vi "运维调试_CODCr.vi"() -> ()   [LabVIEW 2016, in "CODCr库.lvlib"]
uses:
  <vilib>/Utility/miscctls.llb/LVPointTypeDef.ctl
  <vilib>/ptbypt/NI_PtbyPt.lvlib
  <vilib>/Utility/config.llb/NI_LVConfig.lvlib
panel:
  in  "仪器参数":bool
  in  "MB通信方式选择":enum16{"串口", "TCP"}(ring)
  in  "释放串口":bool
  in  "打开串口":bool
  in  "加标回收测试":bool
  in  "平行样测试":bool
  in  "定时启动":bool
  out "COM口":string
  in  "空白测试":bool
  in  "隐藏按钮":bool
  in  "写入消解温度时长":bool
  in  "保存KB值":bool
  in  "标样核查":bool
  out "启动时间":timestamp format="%<%Y/%m/%d %H:%M:%S>T"
  out "主循环次数":i32
  out "status":bool
  out "启动测量模式":T1(ring)
  out "曲线截距B":sgl format="%#_10g"
  out "曲线斜率K":sgl format="%#_10g"
  out "量程上限":sgl
  out "量程下限":sgl
  out "消解时长":u16
  out "消解温度":u16
  out "测量精度":u16
  out "测量结果":sgl
  out "标样参考值":sgl
  out "量程":u16
  out "工作状态":T1(ring)
  out "仪器时间":timestamp format="%<%X\n%x>T"
  out "关键参数区":T2
  out "状态告警区":T3
  out "测量数据区":T4 {"单位" items=["ug/L", "mg/L", "ppm", "mg/m3", "cm", "ppb", "ug/m3", "%", "nmol/mol", "umol/mol", "MPN/L", "MPN/100ml", "ng/m3", "NTU", "无量纲", "ms/cm", "us/cm", "℃", "mV", "万个/L"]}
  out "系统时间":timestamp format="%<%Y/%m/%d %H:%M:%S>T"
  in  "停止":bool
  in  "校时":bool
  in  "标样校准":bool
  in  "空白校准":bool
  in  "零点核查":bool
  in  "跨度核查":bool
  in  "水样测试":bool
  in  "返回":bool
  in  "设置":bool
  # "mg/L"
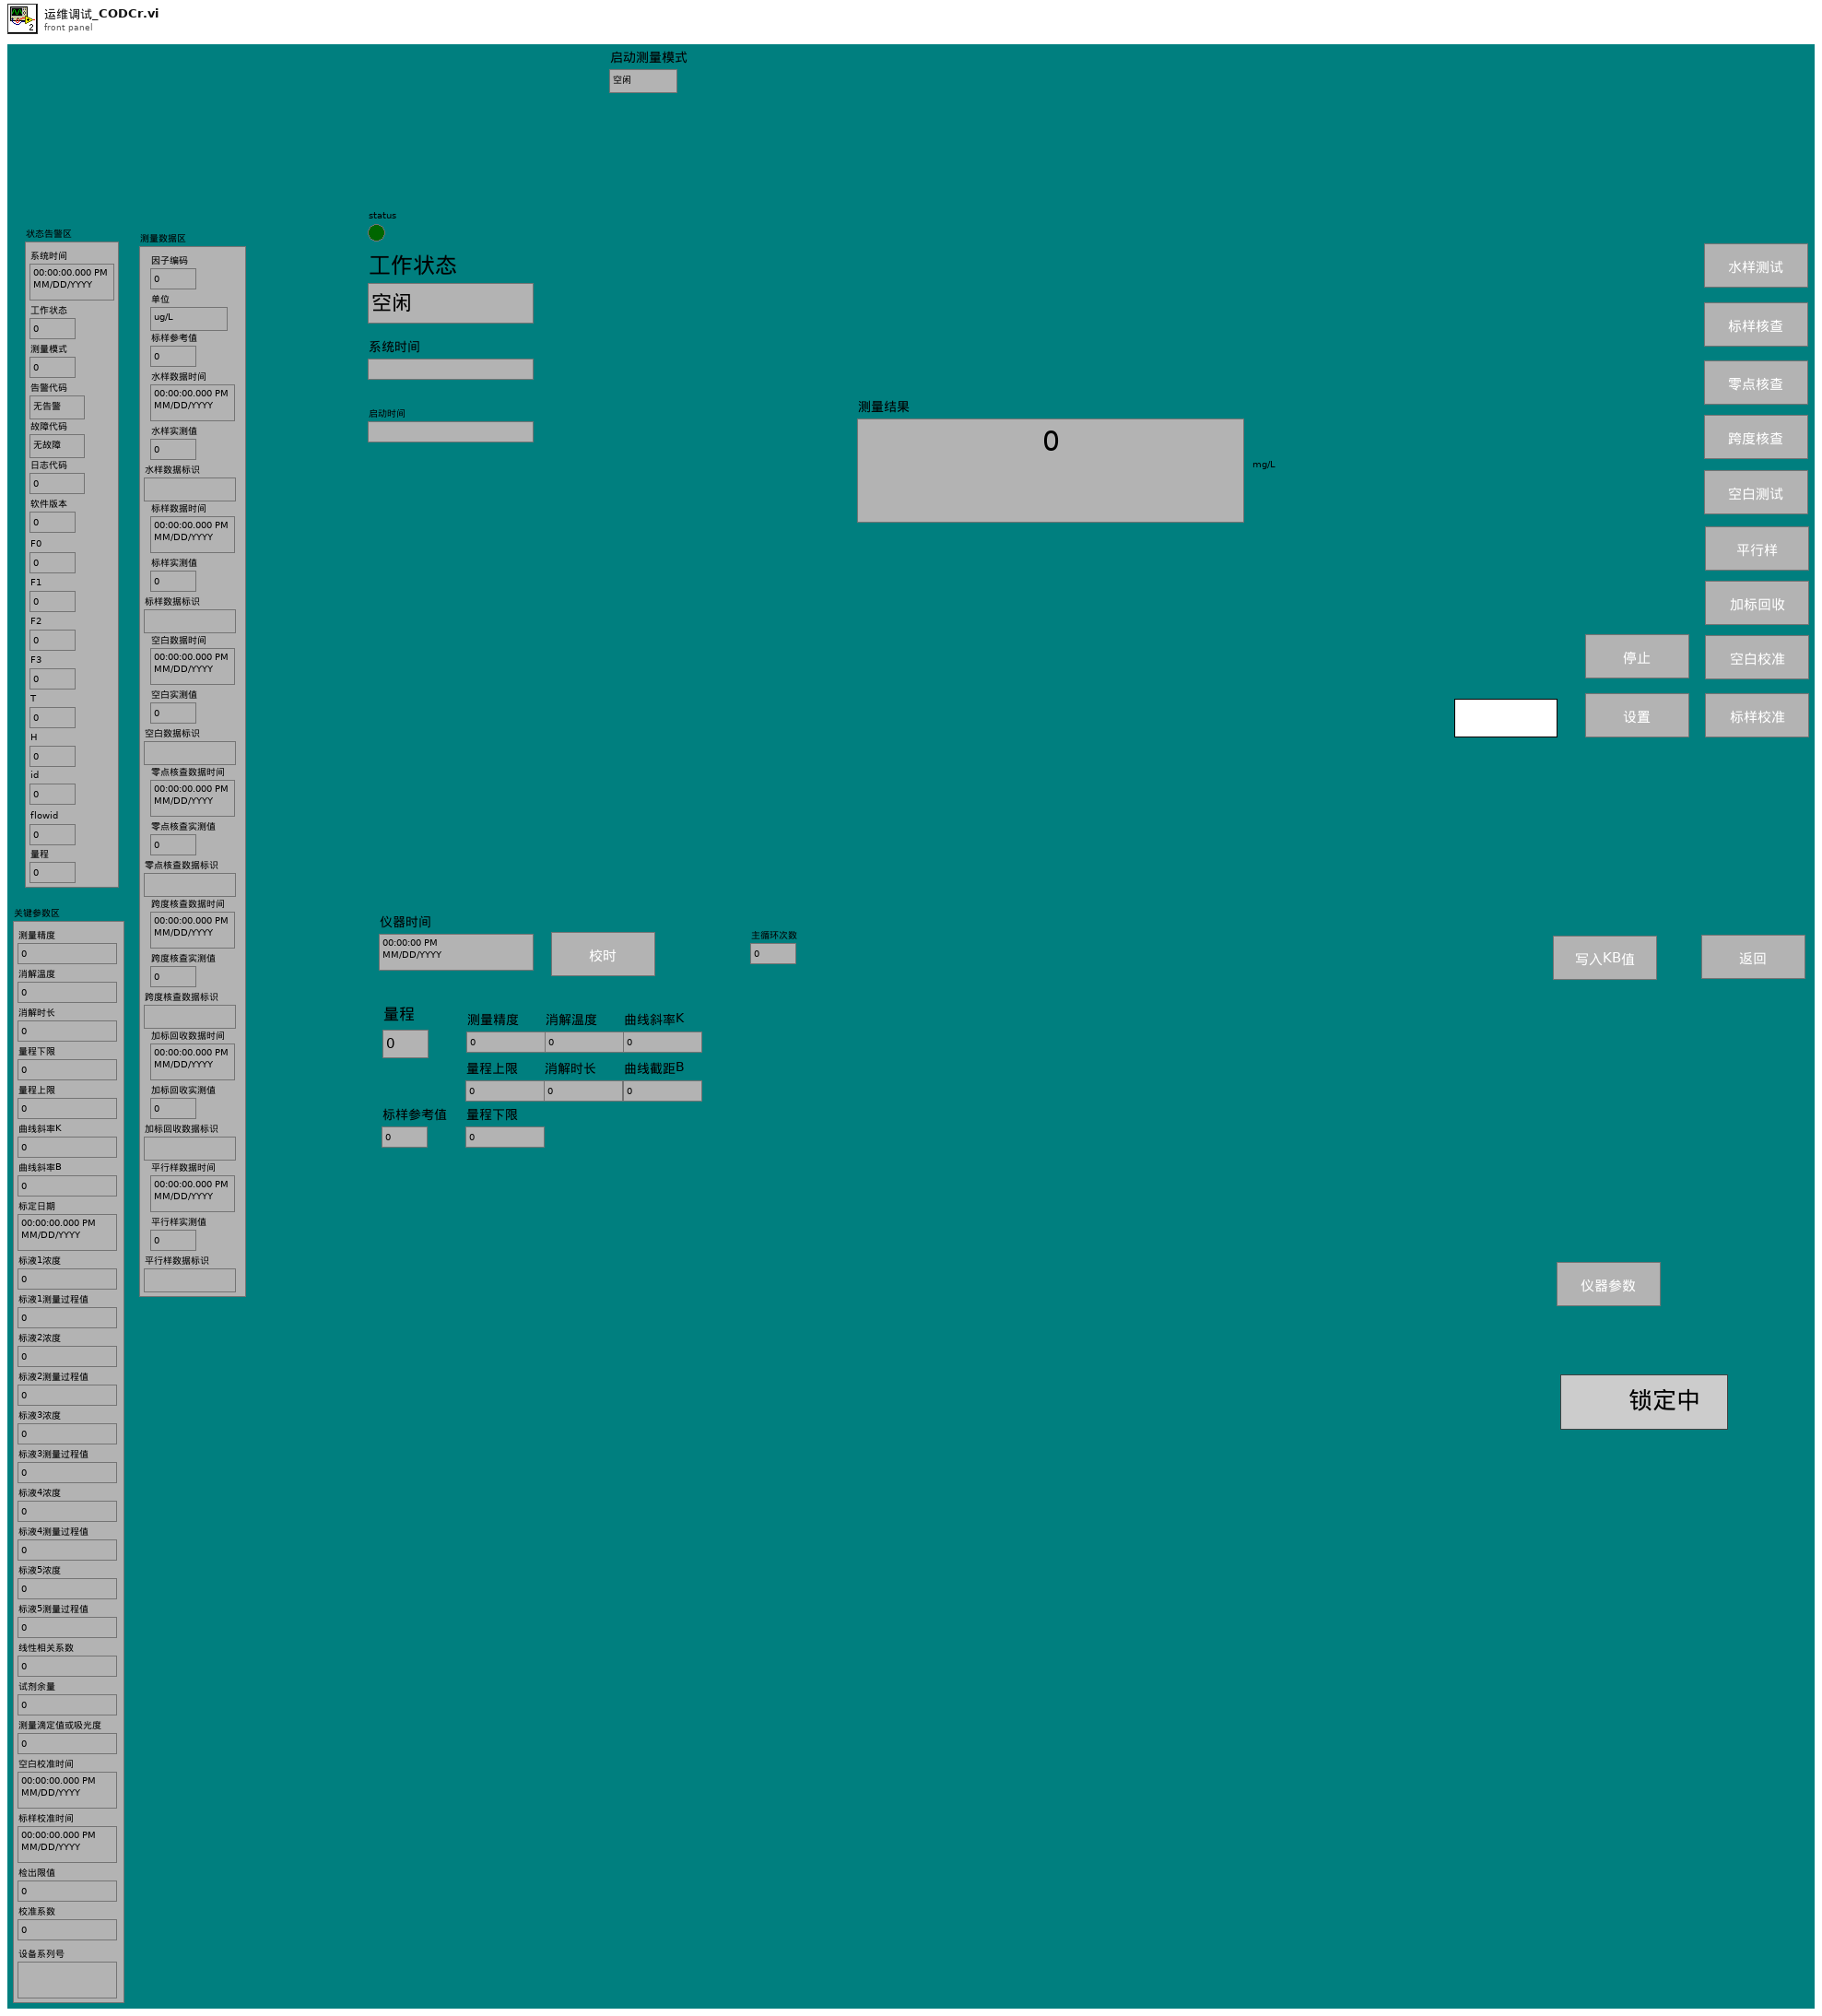
[diagram p1: front panel]
types:
  T1 = enum16{"空闲", "水样测试", "标样核查", "零点核查", "跨度核查", "空白测试", "平行样测试", "加标回收", "空白校准", "标样校准", "初始化（清洗）"}
  T2 = cluster{"测量精度":u16, "消解温度":u16, "消解时长":u16, "量程下限":sgl, "量程上限":sgl, "曲线斜率K":sgl, "曲线斜率B":sgl, "标定日期":timestamp, "标液1浓度":sgl, "标液1测量过程值":sgl, "标液2浓度":sgl, "标液2测量过程值":sgl, "标液3浓度":sgl, "标液3测量过程值":sgl, "标液4浓度":sgl, "标液4测量过程值":sgl, "标液5浓度":sgl, "标液5测量过程值":sgl, "线性相关系数":sgl, "试剂余量":u32, "测量滴定值或吸光度":sgl, "空白校准时间":timestamp, "标样校准时间":timestamp, "检出限值":sgl, "校准系数":sgl, "设备系列号":string}
  T3 = cluster{"系统时间":timestamp, "工作状态":u16, "测量模式":u16, "告警代码":enum16{"无告警", "缺试剂告警", "缺水样告警", "缺蒸馏水告警", "缺标液告警", "仪表漏液告警", "标定异常告警", "超量程告警", "加热异常", "低试剂预警", "超上限告警", "超下限告警", "仪表内部其他异常", "滴定异常告警", "电极异常告警", "量程切换告警", "参数设置告警", "PH电极电位异常", "电导率电极异常", "浊度光度异常", "溶解氧电极异常", "溶解氧光强异常", "温度异常告警", "PH异常告警", "溶解氧异常告警", "电导率异常告警", "浊度异常告警", "叶绿素异常告警", "藻密度异常告警", "蓝绿藻异常告警", "ORP异常告警", "氨氮异常告警", "清洁刷异常告警", "SD卡异常告警", "蓝牙异常告警", "Wifi异常告警", "流程异常告警"}, "故障代码":enum16{"无故障", "电机故障", "温度故障", "通讯故障", "滴定故障"}, "日志代码":u16, "软件版本":u16, "F0":sgl, "F1":sgl, "F2":sgl, "F3":sgl, "T":sgl, "H":sgl, "id":u16, "flowid":u16, "量程":u16}
  T4 = cluster{"因子编码":u32, "单位":u16, "标样参考值":sgl, "水样数据时间":timestamp, "水样实测值":sgl, "水样数据标识":string, "标样数据时间":timestamp, "标样实测值":sgl, "标样数据标识":string, "空白数据时间":timestamp, "空白实测值":sgl, "空白数据标识":string, "零点核查数据时间":timestamp, "零点核查实测值":sgl, "零点核查数据标识":string, "跨度核查数据时间":timestamp, "跨度核查实测值":sgl, "跨度核查数据标识":string, "加标回收数据时间":timestamp, "加标回收实测值":sgl, "加标回收数据标识":string, "平行样数据时间":timestamp, "平行样实测值":sgl, "平行样数据标识":string}
  T5 = cluster{"命令":string, "测量模式":enum16{"水样测量", "标样核查", "零点核查", "跨度核查", "空白测试", "加标回收", "平行样", "校零", "校标"}, "CODCr量程切换":enum32{"H", "L", "AUTO"}}
  T6 = typedef "LVPointTypeDef.ctl" = cluster{"Horizontal":i16, "Vertical":i16}
  T7 = typedef "NI_LVConfig.lvlib/Config Data RefNum.ctl" = refnum<k1>
  T8 = cluster{"运行模式":enum16{"维护模式", "常规模式", "应急模式", "质控模式"}}
  T9 = cluster{"时间标识":timestamp, "监测值":sgl, "单位":u16, "数据标识":string, "因子编码":u32, "标样参考值":sgl, "F0":sgl, "F1":sgl, "F2":sgl, "F3":sgl, "温度":sgl, "湿度":sgl, "量程标识":string, "LastTime":timestamp}
  T10 = cluster{"时间标识":timestamp, "设备":string, "日志信息":string}
  T11 = cluster{"时间标识":timestamp, "参数":string, "日志信息":string, "流程参数":string}
  T12 = enum16{"无告警", "缺试剂告警", "缺水样告警", "缺蒸馏水告警", "缺标液告警", "仪表漏液告警", "标定异常告警", "超量程告警", "加热异常", "低试剂预警", "超上限告警", "超下限告警", "仪表内部其他异常", "滴定异常告警", "电极异常告警", "量程切换告警", "参数设置告警", "PH电极电位异常", "电导率电极异常", "浊度光度异常", "溶解氧电极异常", "溶解氧光强异常", "温度异常告警", "PH异常告警", "溶解氧异常告警", "电导率异常告警", "浊度异常告警", "叶绿素异常告警", "藻密度异常告警", "蓝绿藻异常告警", "ORP异常告警", "氨氮异常告警", "清洁刷异常告警", "SD卡异常告警", "蓝牙异常告警", "Wifi异常告警", "流程异常告警"}
  T13 = cluster{"时间标识":timestamp, "设备":string, "日志信息":string, "流程参数":string}
  T14 = enum16{"水样测量", "标样核查", "零点核查", "跨度核查", "空白测试", "加标回收", "平行样", "校零", "校标"}
  T15 = cluster{"控制命令":enum16{"启动测量", "标样核查", "零点核查", "跨度核查", "空白测试", "平行样测试", "加标回收", "空白校准", "标样校准", "初始化（清洗）", "停止测试", "仪器重启", "校时", "模式设置", "测量间隔设置"}, "周期设置类型":enum16{"定点启动", "间隔启动"}, "定时功能启用":bool, "定时间隔":dbl, "24H周期设置":bool[], "零点核查时间":u16, "跨度核查时间":u16, "质控频次":enum16{"关闭", "每天", "星期一", "星期二", "星期三", "星期四", "星期五", "星期六", "星期日"}}
  T16 = cluster{"测量量程":dbl, "测量精度":dbl, "测量间隔":dbl, "消解温度":dbl, "消解时长":dbl, "空白校准时间":timestamp, "曲线截距":dbl, "曲线斜率":dbl, "测量检出限":dbl, "测量信号值":dbl, "线性相关系数":dbl, "二次多项式系数":dbl, "标样校准时间":timestamp, "稀释倍数":dbl, "三项式系数":dbl, "空白标定系数":dbl, "量程系数":dbl, "F0/ORPA":dbl, "F1/ORPB":dbl, "F2/ORPK":dbl, "F3":dbl, "F4":dbl, "F5":dbl, "F6":dbl, "F7":dbl, "X0/滴定数":dbl, "量程":dbl}
  T17 = cluster{"控制命令":enum16{"启动测量", "标样核查", "零点核查", "跨度核查", "空白测试", "平行样测试", "加标回收", "空白校准", "标样校准", "初始化（清洗）", "停止测试", "仪器重启", "校时", "模式设置", "测量间隔设置"}, "周期设置类型":enum16{"定点启动", "间隔启动"}, "定时功能启用":bool, "定时间隔":dbl, "24H周期设置":bool[], "空白核查时间":u16, "跨度核查时间":u16, "质控频次":enum16{"关闭", "每天", "星期一", "星期二", "星期三", "星期四", "星期五", "星期六", "星期日"}}
  T18 = cluster{"确定":bool, "测量量程":dbl, "测量精度":dbl, "测量间隔":dbl, "消解温度":dbl, "消解时长":dbl, "空白校准时间":timestamp, "曲线截距":dbl, "曲线斜率":dbl, "测量检出限":dbl, "测量信号值":dbl, "线性相关系数":dbl, "二次多项式系数":dbl, "标样校准时间":timestamp, "稀释倍数":dbl, "三项式系数":dbl, "空白标定系数":dbl, "量程系数":dbl, "F0/ORPA":dbl, "F1/ORPB":dbl, "F2/ORPK":dbl, "F3":dbl, "F4":dbl, "F5":dbl, "F6":dbl, "F7":dbl, "X0/滴定数":dbl, "量程":dbl}
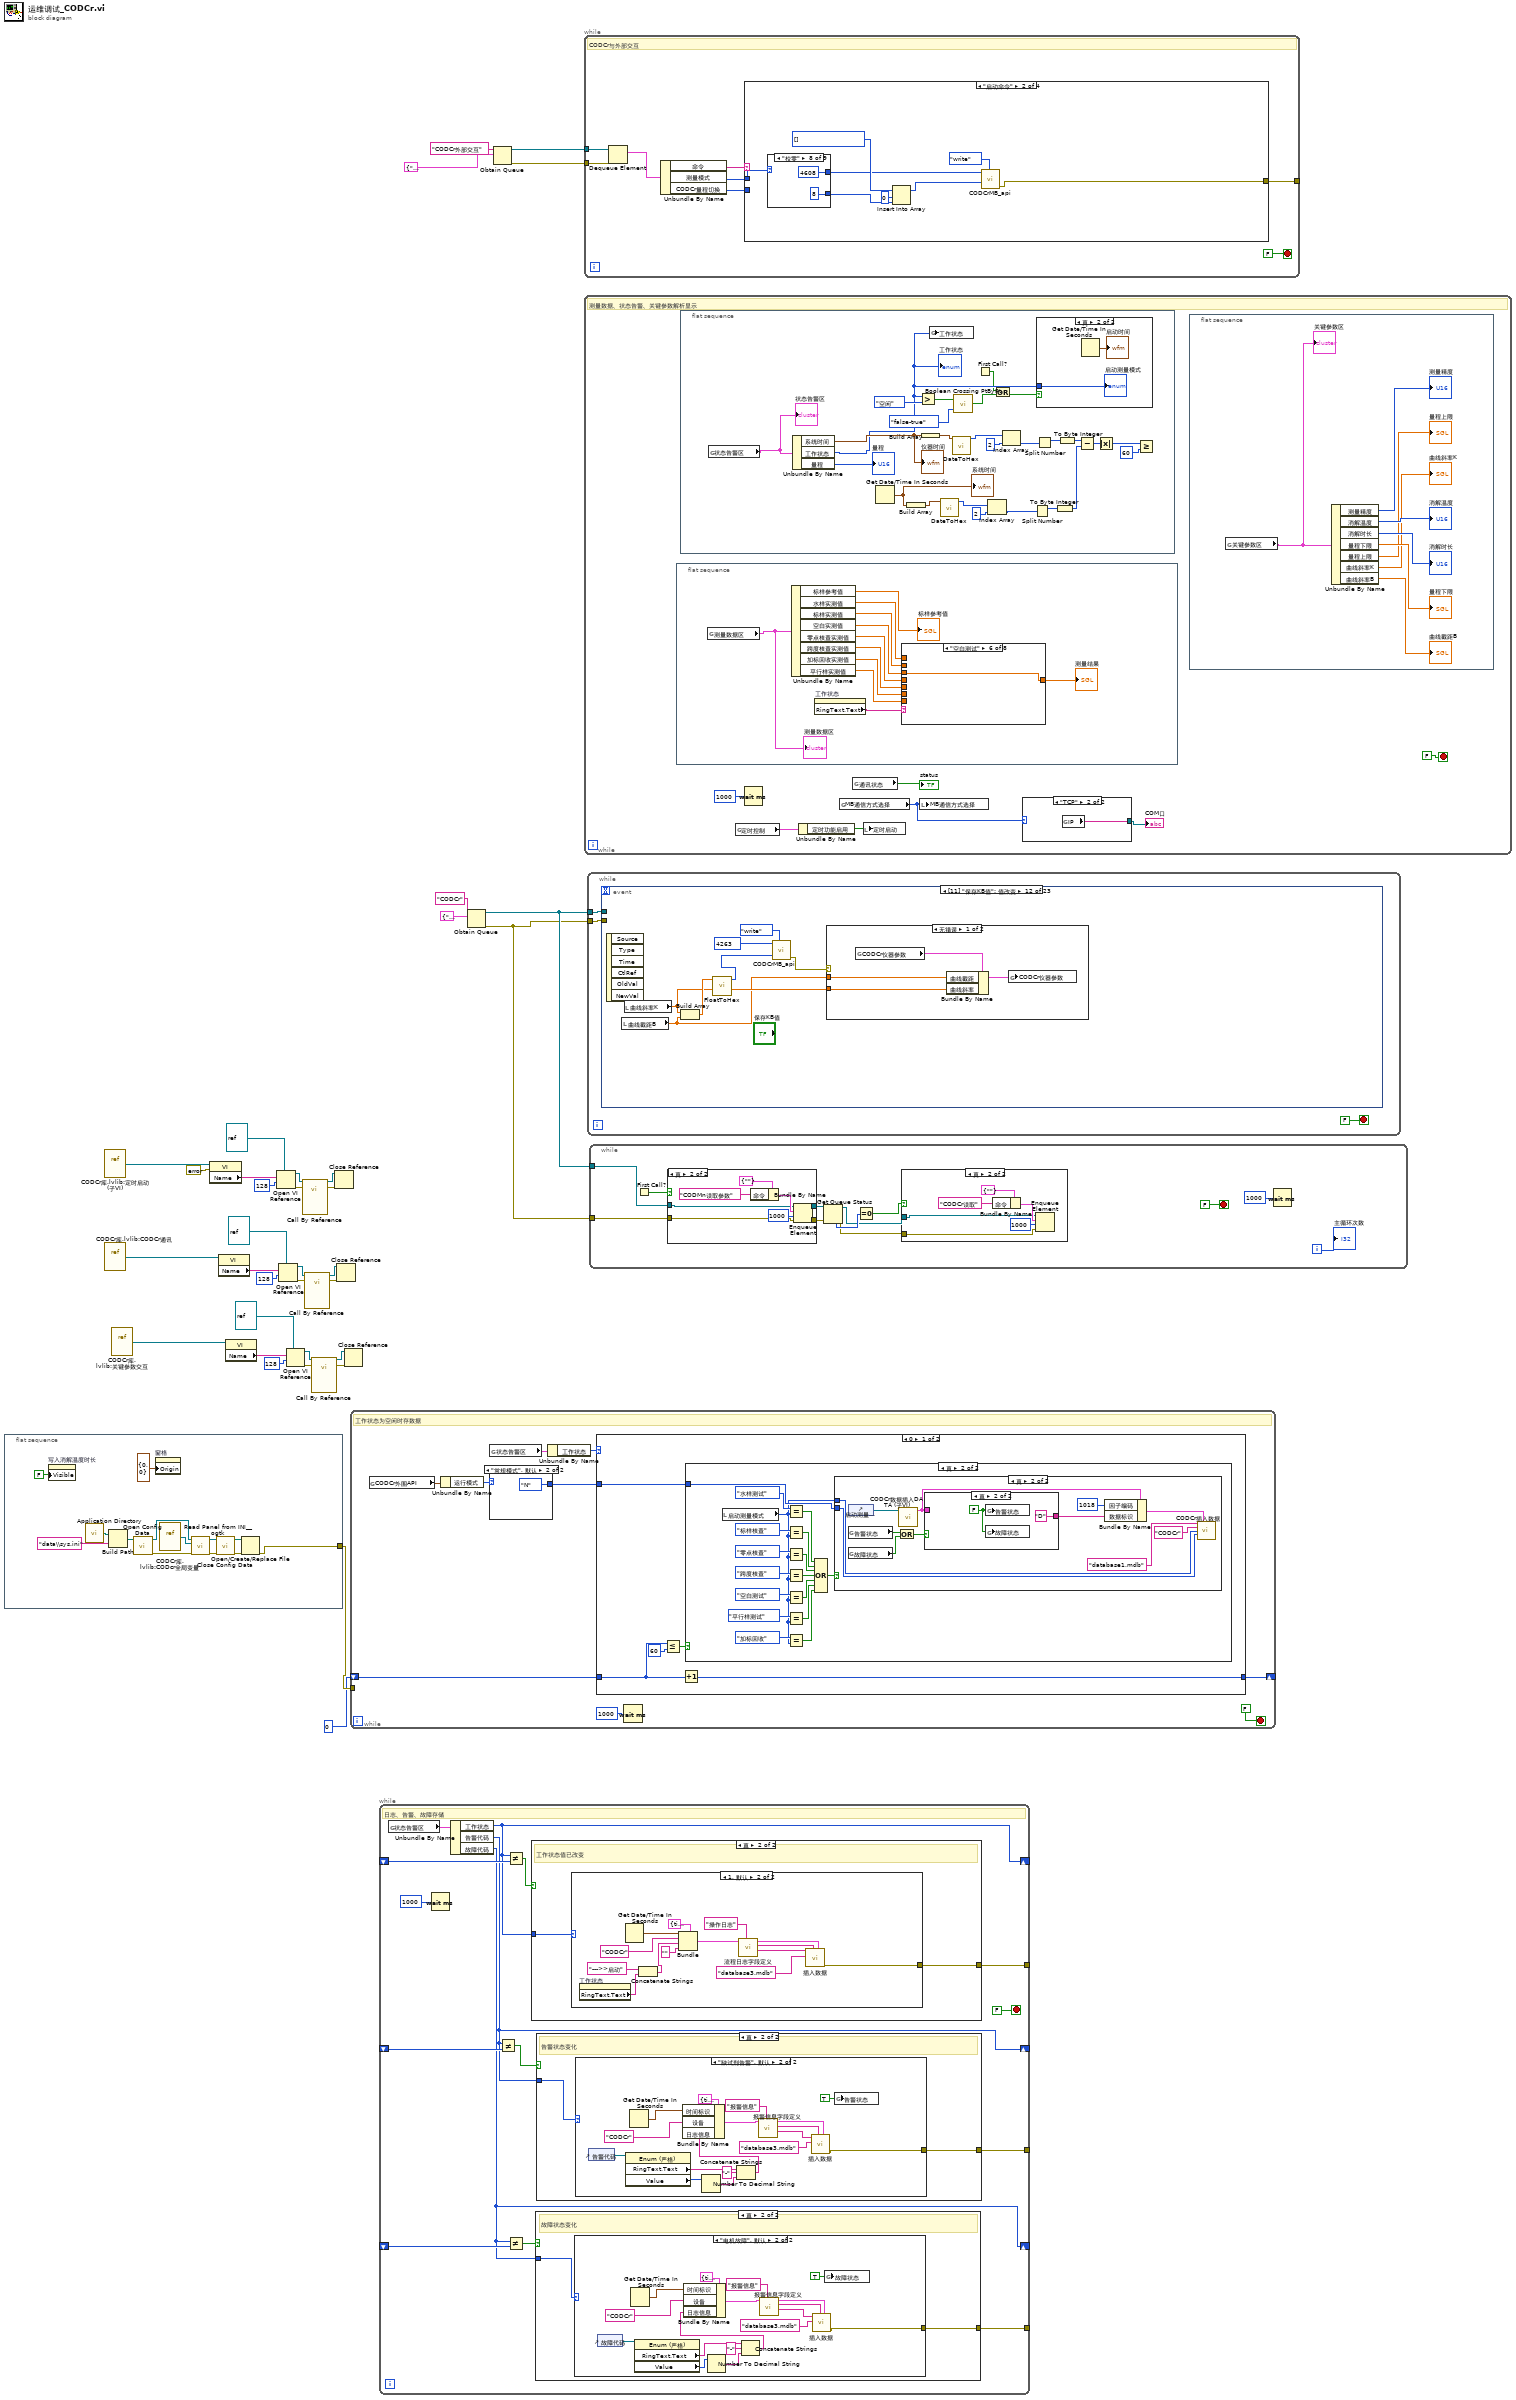
[diagram p0: block diagram]
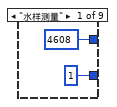
[diagram p5: hidden frame]
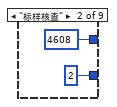
[diagram p6: hidden frame]
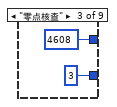
[diagram p7: hidden frame]
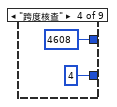
[diagram p8: hidden frame]
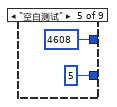
[diagram p9: hidden frame]
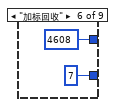
[diagram p10: hidden frame]
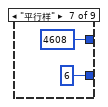
[diagram p11: hidden frame]
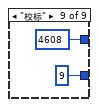
[diagram p12: hidden frame]
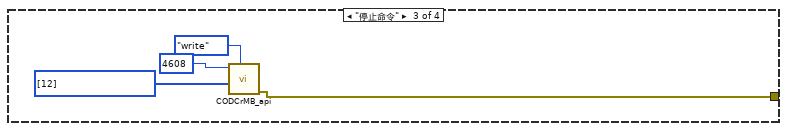
[diagram p13: hidden frame]
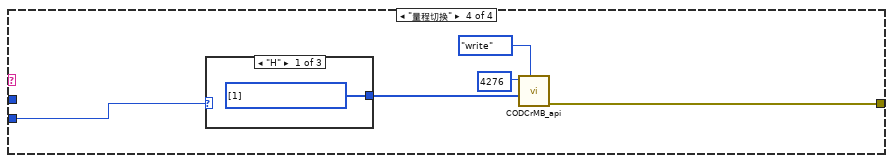
[diagram p14: hidden frame]
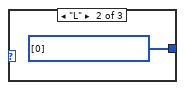
[diagram p15: hidden frame]
diagram:
  n1 = flat-sequence {
    tunnel: [w36] -> w35
    frame #0 {
      n2 = property on="写入消解温度时长" class="Bool"("Visible"=FALSE ("可见")) -> ()  [unwired: 2 in, 2 out]
      n3 = call <vilib>:"Application Directory.vi"() -> ("Application Directory"=w46:path)
      n4 = Build Path(base path=w46, name or relative path="data\\sys.ini" ("名称或相对路径")) -> (appended path=w44:path)
      n5 = call <vilib>:"Open Config Data.vi"("configuration file path"=w44) -> ("error out"=w40:errorcluster, "refnum"=w43:T7)  [unwired: 8 in, 1 out]
      n6 = property on="窗格" class="Pane"("Origin"=T6 {"Horizontal"=0, "Vertical"=0} ("原点")) -> ()  [unwired: 2 in, 2 out]
      n7 = vi-ref "CODCr库.lvlib:CODcr全局变量.vi"() -> (w42:refnum<vi>)
      n8 = call <userlib>:"Read Panel from INI__ogtk.vi"("error in (no error)"=w40, "VI ref"=w42, "refnum"=w43) -> ("error out"=w39:errorcluster, "refnum out"=w41:T7)  [unwired: 7 in]
      n9 = call <vilib>:"Close Config Data.vi"("error in (no error)"=w39, "refnum"=w41) -> ("error out"=w38:errorcluster, "file path"=w37:path)  [unwired: 8 in]
      n10 = Open/Create/Replace File(file path (use dialog)=w37, error in=w38) -> (error out=w36:errorcluster)  [unwired: 4 in, 2 out]
    }
  }
  n11 = vi-ref "CODCr库.lvlib:定时启动 (子VI).vi"() -> (w10:refnum<vi>)
  n12 = vi-ref "CODCr库.lvlib:CODCr通讯.vi"() -> (w27:refnum<vi>)
  n13 = vi-ref "CODCr库.lvlib:关键参数交互.vi"() -> (w9:refnum<vi>)
  n14 = property class="VI"(reference=w10, error in=errorcluster {"status"=FALSE, "code"=0, "source"=""} ("错误输出")) -> ("Name"=w11:string)  [unwired: 2 out]
  n15 = property class="VI"(reference=w27) -> ("Name"=w28:string)  [unwired: 1 in, 2 out]
  n16 = property class="VI"(reference=w9) -> ("Name"=w8:string)  [unwired: 1 in, 2 out]
  n17 = Open VI Reference(type specifier VI Refnum (for type only)=refnum<vi> refnum, vi path=w11, options=128 ("选项")) -> (vi reference=w13:refnum<vi>, error out=w15:errorcluster)  [unwired: 3 in]
  n18 = Open VI Reference(type specifier VI Refnum (for type only)=refnum<vi> refnum, vi path=w28, options=128 ("选项")) -> (vi reference=w30:refnum<vi>, error out=w32:errorcluster)  [unwired: 3 in]
  n19 = Open VI Reference(type specifier VI Refnum (for type only)=refnum<vi> refnum, vi path=w8, options=128 ("选项")) -> (vi reference=w6:refnum<vi>, error out=w4:errorcluster)  [unwired: 3 in]
  n20 = call-by-ref "?"(reference=w13, error in=w15) -> (reference out=w17:refnum<vi>, error out=w16:errorcluster)  [unwired: 12 in]
  n21 = call-by-ref "?"(reference=w30, error in=w32) -> (reference out=w34:refnum<vi>, error out=w33:errorcluster)  [unwired: 12 in]
  n22 = call-by-ref "?"(reference=w6, error in=w4) -> (reference out=w2:refnum<vi>, error out=w3:errorcluster)  [unwired: 12 in]
  n23 = Close Reference(reference=w17, error in (no error)=w16) -> ()  [unwired: 1 out]
  n24 = Close Reference(reference=w34, error in (no error)=w33) -> ()  [unwired: 1 out]
  n25 = Close Reference(reference=w2, error in (no error)=w3) -> ()  [unwired: 1 out]
  n26 = while "While循环" {
    tunnel: w35 -> [_]
    shift-right: [w49] -> _
    shift-left: 0 -> [w50]
    stop <- FALSE stop-if-true
    # "工作状态为空闲时存数据"
    n27 = global read "CODCr外部API.vi" "CODCr外围API"() -> (w53:T8)
    n28 = Unbundle By Name(w53) -> ("运行模式"=w52:enum16{"维护模式", "常规模式", "应急模式", "质控模式"})
    n29 = global read "CODcr全局变量.vi" "状态告警区"() -> (w51:T3)
    n30 = case shown="\"常规模式\", 默认" w52 {
      tunnel: [enum16{"N", "M"}."M" ("数据类型") enum16{"N", "M"}."N" ("数据类型")] -> w54
      frame "维护模式" {
      }
      frame "常规模式", Default {
      }
    }
    n31 = Unbundle By Name(w51) -> ("工作状态"=w55:u16)
    n32 = case shown="0" w55 {
      tunnel: w54 -> [w64 _]
      tunnel: w50 -> [w62 _]
      tunnel: [w63 _] -> w49
      frame 0 {
        n33 = Less Or Equal?(x=w62, y=60) -> (x <= y?=w60:bool)
        n34 = Increment(x=w62) -> (x+1=w63:i32)
        n35 = case shown="真" w60 {
          tunnel: w64 -> [_ w81]
          frame False {
          }
          frame True {
            n36 = local read "启动测量模式"() -> (w73:T1)
            n37 = Equal?(x=T1."水样测试" ("启动测量模式"), y=w73) -> (x = y?=w72:bool)
            n38 = Equal?(x=T1."标样核查" ("启动测量模式"), y=w73) -> (x = y?=w71:bool)
            n39 = Equal?(x=T1."零点核查" ("启动测量模式"), y=w73) -> (x = y?=w70:bool)
            n40 = Equal?(x=T1."跨度核查" ("启动测量模式"), y=w73) -> (x = y?=w69:bool)
            n41 = Equal?(x=T1."空白测试" ("启动测量模式"), y=w73) -> (x = y?=w68:bool)
            n42 = Equal?(x=T1."平行样测试" ("启动测量模式"), y=w73) -> (x = y?=w67:bool)
            n43 = Equal?(x=T1."加标回收" ("启动测量模式"), y=w73) -> (x = y?=w66:bool)
            n44 = Compound Arithmetic op=OR(w72, w71, w70, w69, w68, w67, w66) -> (w65:bool)
            n45 = case shown="真" w65 {
              tunnel: w73 -> [_ w89]
              tunnel: w81 -> [_ w88]
              frame False {
              }
              frame True {
                n46 = control-ref of="启动测量模式"() -> (w93:refnum<vi>)
                n47 = global read "CODcr全局变量.vi" "告警状态"() -> (w86:bool)
                n48 = global read "CODcr全局变量.vi" "故障状态"() -> (w85:bool)
                n49 = Or(x=w86, y=w85) -> (x .or. y?=w84:bool)
                n50 = call "CODCr数据插入DATA (子VI).vi"("Enum输入"=w93) -> ("data"=w83:T9)  [unwired: 10 in]
                n51 = case shown="真" w84 {
                  tunnel: w83 -> [w95 _]
                  tunnel: [w94 "D" ("table")] -> w82
                  frame False {
                    n52 = Unbundle By Name(w95) -> ("数据标识"=w94:string)
                  }
                  frame True {
                    w96 = FALSE ("告警状态")
                    n53 = global write "CODcr全局变量.vi" "告警状态"(w96) -> ()
                    n54 = global write "CODcr全局变量.vi" "故障状态"(w96) -> ()
                  }
                }
                n55 = Bundle By Name(cluster=w83, "因子编码"=u32 1018, "数据标识"=w82) -> (w92:T9)
                n56 = call "CODCr插入数据.vi"("database"="database1.mdb", "data"=w92, "table"="CODCr", "测量模式"=w89, "数据类型"=w88) -> ()  [unwired: 10 in, 1 out]
              }
            }
          }
        }
      }
      frame 1, Default {
      }
    }
    n57 = Wait (ms)(milliseconds to wait=u32 1000 ("等待时间（毫秒）")) -> ()  [unwired: 1 out]
  }
  n58 = while {
    shift-right: [w108] -> _
    shift-left: _ -> [w110]
    tunnel: [w107] -> _
    shift-right: [w103] -> _
    shift-left: _ -> [w104]
    shift-right: [w99] -> _
    shift-left: _ -> [w101]
    tunnel: [w100] -> _
    tunnel: [w98] -> _
    stop <- FALSE stop-if-true
    # "日志、告警、故障存储"
    n59 = global read "CODcr全局变量.vi" "状态告警区"() -> (w106:T3)
    n60 = Wait (ms)(milliseconds to wait=u32 1000 ("等待时间（毫秒）")) -> ()  [unwired: 1 out]
    n61 = Unbundle By Name(w106) -> ("工作状态"=w108:u16, "告警代码"=w103:T12, "故障代码"=w99:enum16{"无故障", "电机故障", "温度故障", "通讯故障", "滴定故障"})
    n62 = Not Equal?(x=w103, y=w104) -> (x != y?=w105:bool)
    n63 = Not Equal?(x=w108, y=w110) -> (x != y?=w109:bool)
    n64 = Not Equal?(x=w99, y=w101) -> (x != y?=w102:bool)
    n65 = case shown="真" w109 {
      tunnel: w108 -> [_ w152]
      tunnel: [_ w151] -> w107
      frame False {
      }
      frame True {
        # "工作状态值已改变"
        n66 = case shown="1, 默认" w152 {
          tunnel: [w153 w168] -> w151
          frame 0 {
            n67 = Get Date/Time In Seconds() -> (seconds since 1Jan1904=w160:timestamp)
            n68 = Bundle(cluster=T11 {"时间标识"=timestamp(0 s since 1904-01-01), "参数"="", "日志信息"="", "流程参数"=""} ("data in"), "时间标识"=w160, "参数"="CODCr" ("table输入"), "日志信息"="--->>结束", "流程参数"="" ("table输入")) -> (w154:T11)
            n69 = call "流程日志字段定义.vi"("table输入"="操作日志", "data in"=w154) -> ("table输出"=w158:string, "columns"=w156:string[], "data out"=w155:T13)  [unwired: 7 in]
            n70 = call "插入数据.vi"("data"=w155, "columns"=w156, "database"="database3.mdb", "table"=w158) -> ("error out"=w153:errorcluster)  [unwired: 7 in]
          }
          frame 1, Default {
            n71 = property on="工作状态" class="Enum (严格)"() -> ("RingText.Text"=w165:string)  [unwired: 2 in, 2 out]
            n72 = Get Date/Time In Seconds() -> (seconds since 1Jan1904=w175:timestamp)
            n73 = Concatenate Strings("--->>启动" ("日志信息"), w165) -> (w166:string)
            n74 = Bundle(cluster=T11 {"时间标识"=timestamp(0 s since 1904-01-01), "参数"="", "日志信息"="", "流程参数"=""} ("data in"), "时间标识"=w175, "参数"="CODCr" ("table输入"), "日志信息"=w166, "流程参数"="" ("table输入")) -> (w174:T11)
            n75 = call "流程日志字段定义.vi"("table输入"="操作日志", "data in"=w174) -> ("table输出"=w172:string, "columns"=w170:string[], "data out"=w169:T13)  [unwired: 7 in]
            n76 = call "插入数据.vi"("data"=w169, "columns"=w170, "database"="database3.mdb", "table"=w172) -> ("error out"=w168:errorcluster)  [unwired: 7 in]
          }
        }
      }
    }
    n77 = case shown="真" w102 {
      tunnel: w99 -> [_ w114]
      tunnel: [_ w113] -> w98
      frame False {
      }
      frame True {
        # "故障状态变化"
        n78 = case shown="\"电机故障\", 默认" w114 {
          tunnel: [_ w121] -> w113
          frame "无故障" {
            # "无告警"
          }
          frame "电机故障", Default {
            n79 = control-ref of="故障代码"() -> (w131:refnum<vi>)
            n80 = Get Date/Time In Seconds() -> (seconds since 1Jan1904=w129:timestamp)
            n81 = property class="Enum (严格)"(reference=w131) -> ("RingText.Text"=w118:string, "Value"=w119:enum16{"无故障", "电机故障", "温度故障", "通讯故障", "滴定故障"})  [unwired: 1 in, 2 out]
            n82 = Number To Decimal String(number=w119) -> (decimal integer string=w116:string)  [unwired: 1 in]
            n83 = Concatenate Strings(w118, "-" ("字符串"), w116) -> (w117:string)
            n84 = Bundle By Name(cluster=T10 {"时间标识"=timestamp(0 s since 1904-01-01), "设备"="", "日志信息"=""} ("data in"), "时间标识"=w129, "设备"="CODCr" ("table输入"), "日志信息"=w117) -> (w128:T10)
            n85 = call "报警信息字段定义.vi"("table输入"="报警信息", "data in"=w128) -> ("table输出"=w123:string, "columns"=w122:string[], "data out"=w125:T10)  [unwired: 7 in]
            n86 = call "插入数据.vi"("data"=w125, "columns"=w122, "database"="database3.mdb", "table"=w123) -> ("error out"=w121:errorcluster)  [unwired: 7 in]
            n87 = global write "CODcr全局变量.vi" "故障状态"(TRUE ("告警状态")) -> ()
          }
        }
      }
    }
    n88 = case shown="真" w105 {
      tunnel: w103 -> [_ w133]
      tunnel: [_ w132] -> w100
      frame False {
      }
      frame True {
        # "告警状态变化"
        n89 = case shown="\"缺试剂告警\", 默认" w133 {
          tunnel: [_ w143] -> w132
          frame "无告警" {
            # "无告警"
          }
          frame "缺试剂告警", Default {
            n90 = control-ref of="告警代码"() -> (w140:refnum<vi>)
            n91 = property class="Enum (严格)"(reference=w140) -> ("RingText.Text"=w138:string, "Value"=w137:T12)  [unwired: 1 in, 2 out]
            n92 = Get Date/Time In Seconds() -> (seconds since 1Jan1904=w142:timestamp)
            n93 = Number To Decimal String(number=w137) -> (decimal integer string=w134:string)  [unwired: 1 in]
            n94 = Concatenate Strings(w138, "-" ("字符串"), w134) -> (w136:string)
            n95 = Bundle By Name(cluster=T10 {"时间标识"=timestamp(0 s since 1904-01-01), "设备"="", "日志信息"=""} ("data in"), "时间标识"=w142, "设备"="CODCr" ("table输入"), "日志信息"=w136) -> (w144:T10)
            n96 = call "报警信息字段定义.vi"("table输入"="报警信息", "data in"=w144) -> ("table输出"=w149:string, "columns"=w150:string[], "data out"=w147:T10)  [unwired: 7 in]
            n97 = call "插入数据.vi"("data"=w147, "columns"=w150, "database"="database3.mdb", "table"=w149) -> ("error out"=w143:errorcluster)  [unwired: 7 in]
            n98 = global write "CODcr全局变量.vi" "告警状态"(TRUE ("告警状态")) -> ()
          }
        }
      }
    }
  }
  n99 = Obtain Queue(name (unnamed)="CODCr" ("名称（未命名）"), element data type=cluster{"命令":string} {"命令"="启用模块"} ("元素")) -> (queue out=w20:refnum<queue>, error out=w19:errorcluster)  [unwired: 3 in, 1 out]
  n100 = Obtain Queue(name (unnamed)="CODCr外部交互" ("名称（未命名）"), element data type=T5 {"命令"="启动命令", "测量模式"=enum."水样测量", "CODCr量程切换"=enum."AUTO"} ("元素")) -> (queue out=w22:refnum<queue>, error out=w21:errorcluster)  [unwired: 3 in, 1 out]
  n101 = while {
    tunnel: w22 -> [w184]
    tunnel: w21 -> [w183]
    tunnel: [w179] -> _
    stop <- FALSE stop-if-true
    # "CODCr与外部交互"
    n102 = Dequeue Element(queue=w184, error in (no error)=w183) -> (element=w185:T5)  [unwired: 1 in, 3 out]
    n103 = Unbundle By Name(w185) -> ("命令"=w182:string, "测量模式"=w181:T14, "CODCr量程切换"=w180:enum32{"H", "L", "AUTO"})
    n104 = case shown="\"启动命令\"" w182 {
      tunnel: w181 -> [_ w188 _ _]
      tunnel: w180 -> [_ _ _ w218]
      tunnel: [_ w187 w213 w217] -> w179
      frame "假", Default {
      }
      frame "启动命令" {
        n105 = case shown="\"校零\"" w188 {
          tunnel: [u16 4608 ("address") u16 4608 ("address") u16 4608 ("address") u16 4608 ("address") u16 4608 ("address") u16 4608 ("address") u16 4608 ("address") u16 4608 ("address") u16 4608 ("address")] -> w190
          tunnel: [u16 1 ("address") u16 2 ("address") u16 3 ("address") u16 4 ("address") u16 5 ("address") u16 7 ("address") u16 6 ("address") u16 8 ("address") u16 9 ("address")] -> w194
          frame "水样测量" {
          }
          frame "标样核查" {
          }
          frame "零点核查" {
          }
          frame "跨度核查" {
          }
          frame "空白测试" {
          }
          frame "加标回收" {
          }
          frame "平行样" {
          }
          frame "校零" {
          }
          frame "校标" {
          }
        }
        n106 = Insert Into Array(array=u16[] [] ("values"), index=0 ("索引"), new element=w194) -> (w189:u16[])
        n107 = call "CODCrMB_api.vi"("STEP"=enum16{"open", "read", "write", "close"}."write", "values"=w189, "starting address"=w190) -> ("error out"=w187:errorcluster)  [unwired: 6 in, 2 out]
      }
      frame "停止命令" {
        n108 = call "CODCrMB_api.vi"("STEP"=enum16{"open", "read", "write", "close"}."write", "values"=u16[] [12], "starting address"=u16 4608) -> ("error out"=w213:errorcluster)  [unwired: 6 in, 2 out]
      }
      frame "量程切换" {
        n109 = case shown="\"H\"" w218 {
          tunnel: [u16[] [1] ("values") u16[] [0] ("values") _] -> w221
          frame "H" {
          }
          frame "L" {
          }
          frame "AUTO", Default {
          }
        }
        n110 = call "CODCrMB_api.vi"("STEP"=enum16{"open", "read", "write", "close"}."write", "values"=w221, "starting address"=u16 4276) -> ("error out"=w217:errorcluster)  [unwired: 6 in, 2 out]
      }
    }
  }
  n111 = while {
    stop <- FALSE stop-if-true
    # "测量数据、状态告警、关键参数解析显示"
    n112 = flat-sequence {
      frame #0 {
        n113 = global read "CODcr全局变量.vi" "测量数据区"() -> (w269:T4)
        "测量数据区" <- w269
        n114 = Unbundle By Name(w269) -> ("标样参考值"=→"标样参考值":sgl, "水样实测值"=w277:sgl, "标样实测值"=w275:sgl, "空白实测值"=w272:sgl, "零点核查实测值"=w274:sgl, "跨度核查实测值"=w273:sgl, "加标回收实测值"=w270:sgl, "平行样实测值"=w271:sgl)
        n115 = property on="工作状态" class="Enum (严格)"() -> ("RingText.Text"=w278:string)  [unwired: 2 in, 2 out]
        n116 = case shown="\"空白测试\"" w278 {
          tunnel: w277 -> [_ w281 _ _ _ _ _ _]
          tunnel: [w280 w281 w282 w283 w284 w285 w286 w287] -> w276
          tunnel: w275 -> [_ _ w282 _ _ _ _ _]
          tunnel: w274 -> [_ _ _ w283 _ _ _ _]
          tunnel: w273 -> [_ _ _ _ w284 _ _ _]
          tunnel: w272 -> [_ _ _ _ _ w285 _ _]
          tunnel: w271 -> [_ _ _ _ _ _ w286 _]
          tunnel: w270 -> [_ _ _ _ _ _ _ w287]
          frame "空闲", Default {
            n117 = local read "测量结果"() -> (w280:sgl)
          }
          frame "水样测试" {
          }
          frame "标样核查" {
          }
          frame "零点核查" {
          }
          frame "跨度核查" {
          }
          frame "空白测试" {
          }
          frame "平行样测试" {
          }
          frame "加标回收" {
          }
        }
        "测量结果" <- w276
      }
    }
    n118 = flat-sequence {
      frame #0 {
        n119 = global read "CODcr全局变量.vi" "状态告警区"() -> (w241:T3)
        "状态告警区" <- w241
        n120 = Unbundle By Name(w241) -> ("系统时间"=w253:timestamp, "工作状态"=w244:u16, "量程"=→"量程":u16)
        "仪器时间" <- w253
        "工作状态" <- w244
        n121 = Get Date/Time In Seconds() -> (seconds since 1Jan1904=w254:timestamp)
        "系统时间" <- w254
        n122 = Build Array(w254) -> (w248:timestamp[])
        n123 = Greater?(x=w244, y=T1."空闲") -> (0:w252:bool)
        n124 = Build Array(w253) -> (w247:timestamp[])
        n125 = global write "CODcr全局变量.vi" "工作状态"(w244) -> ()
        n126 = call "DateToHex.vi"("DATE"=w248) -> ("数组"=w245:u16[])  [unwired: 10 in]
        n127 = call "DateToHex.vi"("DATE"=w247) -> ("数组"=w246:u16[])  [unwired: 10 in]
        n128 = call <vilib>:"Boolean Crossing PtByPt.vi"("direction"=enum16{"either", "false-true", "true-false"}."false-true", "input"=w252) -> ("crossing"=w251:bool)  [unwired: 1 in]
        n129 = First Call?() -> (First Call?: T/F=w242:bool)
        n130 = Index Array(array=w245, index=2 ("索引")) -> (element=w256:u16)
        n131 = Or(x=w242, y=w251) -> (x .or. y?=w243:bool)
        n132 = Index Array(array=w246, index=2 ("索引")) -> (element=w257:u16)
        n133 = Split Number(x=w256) -> (hi(x)=w259:u8)  [unwired: 1 out]
        n134 = Split Number(x=w257) -> (hi(x)=w262:u8)  [unwired: 1 out]
        n135 = case shown="真" w243 {
          tunnel: w244 -> [_ w267]
          frame False {
          }
          frame True {
            n136 = Get Date/Time In Seconds() -> (seconds since 1Jan1904=→"启动时间":timestamp)
            "启动测量模式" <- w267
          }
        }
        n137 = To Byte Integer(number=w259) -> (8bit integer=w260:i8)
        n138 = To Byte Integer(number=w262) -> (8bit integer=w263:i8)
        n139 = Subtract(x=w263, y=w260) -> (x-y=w261:i8)
        n140 = Absolute Value(x=w261) -> (abs(x)=w264:i8)
        n141 = Greater Or Equal?(x=w264, y=i8 60) -> ()  [unwired: 1 out]
      }
    }
    n142 = global read "CODcr全局变量.vi" "定时控制"() -> (w225:T15)
    n143 = Wait (ms)(milliseconds to wait=u32 1000 ("等待时间（毫秒）")) -> ()  [unwired: 1 out]
    n144 = Unbundle By Name(w225) -> ("定时功能启用"=w224:bool)
    n145 = global read "CODcr全局变量.vi" "MB通信方式选择"() -> (w226:enum16{"串口", "TCP"})
    n146 = global read "CODcr全局变量.vi" "通讯状态"() -> (→"status":bool)
    n147 = local write "定时启动"(w224) -> ()
    n148 = local write "MB通信方式选择"(w226) -> ()
    n149 = case shown="\"TCP\"" w226 {
      tunnel: [w231 w232] -> w227
      frame "串口", Default {
        n150 = global read "CODcr全局变量.vi" "VISA Resource"() -> (w231:refnum<visa-resource-name>)
      }
      frame "TCP" {
        n151 = global read "CODcr全局变量.vi" "IP"() -> (w232:string)
      }
    }
    "COM口" <- w227
    n152 = flat-sequence {
      frame #0 {
        n153 = global read "CODcr全局变量.vi" "关键参数区"() -> (w233:T2)
        "关键参数区" <- w233
        n154 = Unbundle By Name(w233) -> ("测量精度"=→"测量精度":u16, "消解温度"=→"消解温度":u16, "消解时长"=→"消解时长":u16, "量程下限"=→"量程下限":sgl, "量程上限"=→"量程上限":sgl, "曲线斜率K"=→"曲线斜率K":sgl, "曲线斜率B"=→"曲线截距B":sgl)
      }
    }
  }
  n155 = while {
    tunnel: w20 -> [w289]
    tunnel: w19 -> [w288]
    stop <- FALSE stop-if-true
    n156 = event shown="[11] \"保存KB值\": 值改变" {
      selector: _ -> [_ _ _ _ _ _ _ _ _ _ _ _ _ _ _ _ _ _ _ _ _ _ _]
      dyn-events: _ -> [_ _ _ _ _ _ _ _ _ _ _ _ _ _ _ _ _ _ _ _ _ _ _]
      timeout: _ -> [_ _ _ _ _ _ _ _ _ _ _ _ _ _ _ _ _ _ _ _ _ _ _]
      tunnel: w289 -> [_ _ _ _ _ _ _ _ _ _ _ _ _ _ w405 w422 _ _ _ w460 _ _ _]
      tunnel: w288 -> [_ _ _ _ _ _ _ _ _ _ _ _ _ _ w404 w421 _ _ _ w459 _ _ _]
      event Timeout {
        n157 = event-data() -> ()  [unwired: 1 in, 2 out]
      }
      event "水样测试": Value Change {
        n158 = event-data() -> ()  [unwired: 1 in, 6 out]
        n159 = local write "启动测量模式"(T1."水样测试" ("启动测量模式")) -> ()
        n160 = call "CODCrMB_api.vi"("STEP"=enum16{"open", "read", "write", "close"}."write", "values"=u16[] [1], "starting address"=u16 4608) -> ()  [unwired: 6 in, 3 out]
      }
      event "标样核查": Value Change {
        n161 = event-data() -> ()  [unwired: 1 in, 6 out]
        n162 = local write "启动测量模式"(T1."标样核查" ("启动测量模式")) -> ()
        n163 = call "CODCrMB_api.vi"("STEP"=enum16{"open", "read", "write", "close"}."write", "values"=u16[] [2], "starting address"=u16 4608) -> ()  [unwired: 6 in, 3 out]
      }
      event "零点核查": Value Change {
        n164 = event-data() -> ()  [unwired: 1 in, 6 out]
        n165 = local write "启动测量模式"(T1."零点核查" ("启动测量模式")) -> ()
        n166 = call "CODCrMB_api.vi"("STEP"=enum16{"open", "read", "write", "close"}."write", "values"=u16[] [3], "starting address"=u16 4608) -> ()  [unwired: 6 in, 3 out]
      }
      event "跨度核查": Value Change {
        n167 = event-data() -> ()  [unwired: 1 in, 6 out]
        n168 = local write "启动测量模式"(T1."跨度核查" ("启动测量模式")) -> ()
        n169 = call "CODCrMB_api.vi"("STEP"=enum16{"open", "read", "write", "close"}."write", "values"=u16[] [4], "starting address"=u16 4608) -> ()  [unwired: 6 in, 3 out]
      }
      event "空白测试": Value Change {
        n170 = event-data() -> ()  [unwired: 1 in, 6 out]
        n171 = local write "启动测量模式"(T1."空白测试" ("启动测量模式")) -> ()
        n172 = call "CODCrMB_api.vi"("STEP"=enum16{"open", "read", "write", "close"}."write", "values"=u16[] [5], "starting address"=u16 4608) -> ()  [unwired: 6 in, 3 out]
      }
      event "平行样测试": Value Change {
        n173 = event-data() -> ()  [unwired: 1 in, 6 out]
        n174 = local write "启动测量模式"(T1."平行样测试" ("启动测量模式")) -> ()
        n175 = call "CODCrMB_api.vi"("STEP"=enum16{"open", "read", "write", "close"}."write", "values"=u16[] [6], "starting address"=u16 4608) -> ()  [unwired: 6 in, 3 out]
      }
      event "加标回收测试": Value Change {
        n176 = event-data() -> ()  [unwired: 1 in, 6 out]
        n177 = local write "启动测量模式"(T1."加标回收" ("启动测量模式")) -> ()
        n178 = call "CODCrMB_api.vi"("STEP"=enum16{"open", "read", "write", "close"}."write", "values"=u16[] [7], "starting address"=u16 4608) -> ()  [unwired: 6 in, 3 out]
      }
      event "空白校准": Value Change {
        n179 = event-data() -> ()  [unwired: 1 in, 6 out]
        n180 = local write "启动测量模式"(T1."空白校准" ("启动测量模式")) -> ()
        n181 = call "CODCrMB_api.vi"("STEP"=enum16{"open", "read", "write", "close"}."write", "values"=u16[] [8], "starting address"=u16 4608) -> ()  [unwired: 6 in, 3 out]
      }
      event "标样校准": Value Change {
        n182 = event-data() -> ()  [unwired: 1 in, 6 out]
        n183 = local write "启动测量模式"(T1."标样校准" ("启动测量模式")) -> ()
        n184 = call "CODCrMB_api.vi"("STEP"=enum16{"open", "read", "write", "close"}."write", "values"=u16[] [9], "starting address"=u16 4608) -> ()  [unwired: 6 in, 3 out]
      }
      event "停止": Value Change {
        n185 = event-data() -> ()  [unwired: 1 in, 6 out]
        n186 = Two Button Dialog(message="确认是否停止？" ("消息"), 1:"否" ("F按钮名称（“取消”）"), 2:"是" ("T按钮名称（“确定”）")) -> (T button?=w327:bool)
        n187 = case shown="真" w327 {
          frame False {
          }
          frame True {
            n188 = Obtain Notifier(name (unnamed)="CODCr" ("名称（未命名）"), notification data type=FALSE) -> (notifier out=w335:refnum<notifier>, error out=w333:errorcluster)  [unwired: 2 in, 1 out]
            n189 = call "CODCrMB_api.vi"("STEP"=enum16{"open", "read", "write", "close"}."write", "values"=u16[] [12], "starting address"=u16 4608) -> ()  [unwired: 6 in, 3 out]
            n190 = Send Notification(notification=TRUE ("通知"), notifier=w335, error in (no error)=w333) -> (notifier out=w332:refnum<notifier>, error out=w331:errorcluster)
            n191 = Release Notifier(notifier=w332, error in (no error)=w331) -> ()  [unwired: 1 in, 3 out]
          }
        }
      }
      event "保存KB值": Value Change {
        n192 = event-data() -> ()  [unwired: 1 in, 6 out]
        n193 = local read "曲线截距B"() -> (w341:sgl)
        n194 = local read "曲线斜率K"() -> (w342:sgl)
        n195 = Build Array(w342, w341) -> (w347:sgl[])
        n196 = call "FloatToHex.vi"("浮点数"=w347) -> ("DCBA整形输出"=w344:u16[])  [unwired: 10 in]
        n197 = call "CODCrMB_api.vi"("STEP"=enum16{"open", "read", "write", "close"}."write", "values"=w344, "starting address"=u16 4263) -> ("error out"=w343:errorcluster)  [unwired: 6 in, 2 out]
        n198 = case shown="无错误" w343 {
          tunnel: w342 -> [w349 _]
          tunnel: w341 -> [w348 _]
          frame No Error {
            n199 = global read "CODcr全局变量.vi" "CODCr仪器参数"() -> (w351:T16)
            n200 = Bundle By Name(cluster=w351, "曲线截距"=w348, "曲线斜率"=w349) -> (w350:T16)
            n201 = global write "CODcr全局变量.vi" "CODCr仪器参数"(w350) -> ()
          }
          frame Error {
          }
        }
      }
      event "定时启动": Value Change {
        n202 = event-data() -> ()  [unwired: 1 in, 6 out]
        n203 = flat-sequence {
          frame #0 {
            n204 = global read "CODcr全局变量.vi" "定时控制"() -> (w353:T15)
            n205 = call "周期设置.vi"("定时控制输入"=w353) -> ("定时控制输出"=w352:T17)  [unwired: 10 in]
            n206 = global write "CODcr全局变量.vi" "定时控制"(w352) -> ()
          }
          frame #1 {
            n207 = call <vilib>:"Application Directory.vi"() -> ("Application Directory"=w367:path)
            n208 = Build Path(base path=w367, name or relative path="data\\sys.ini" ("名称或相对路径")) -> (appended path=w365:path)
            n209 = call <vilib>:"Open Config Data.vi"("configuration file path"=w365) -> ("error out"=w361:errorcluster, "refnum"=w364:T7)  [unwired: 8 in, 1 out]
            n210 = vi-ref "CODCr库.lvlib:CODcr全局变量.vi"() -> (w363:refnum<vi>)
            n211 = call <userlib>:"Write Panel to INI__ogtk.vi"("error in (no error)"=w361, "VI ref"=w363, "refnum"=w364) -> ("error out"=w360:errorcluster, "refnum out"=w362:T7)  [unwired: 7 in]
            n212 = call <vilib>:"Close Config Data.vi"("error in (no error)"=w360, "refnum"=w362) -> ("error out"=w355:errorcluster, "file path"=w354:path)  [unwired: 8 in]
            n213 = Open/Create/Replace File(file path (use dialog)=w354, error in=w355) -> (refnum out=w358:refnum<file>, error out=w359:errorcluster)  [unwired: 4 in, 1 out]
            n214 = Flush File(refnum=w358, error in=w359) -> (refnum out=w357:refnum<file>, error out=w356:errorcluster)
            n215 = Close File(refnum=w357, error in=w356) -> ()  [unwired: 2 out]
          }
        }
      }
      event "仪器参数": Value Change {
        n216 = event-data() -> ()  [unwired: 1 in, 6 out]
        n217 = global read "CODcr全局变量.vi" "CODCr仪器参数"() -> (w369:T16)
        n218 = call "仪器参数设置.vi"("氨氮仪器参数"=w369) -> ("仪器参数设置输出"=w368:T18)  [unwired: 10 in]
        n219 = Unbundle By Name(w368) -> ("确定"=w370:bool)
        n220 = case shown="真" w370 {
          tunnel: w369 -> [_ w372]
          tunnel: w368 -> [_ w371]
          frame False {
          }
          frame True {
            n221 = flat-sequence {
              tunnel: w372 -> [w389]
              tunnel: w371 -> [w388]
              frame #0 {
                n222 = Unbundle By Name(w388) -> ("测量量程"=w387:dbl, "测量精度"=w386:dbl, "测量间隔"=w385:dbl, "消解温度"=w384:dbl, "消解时长"=w383:dbl, "空白校准时间"=w382:timestamp, "曲线截距"=w381:dbl, "曲线斜率"=w380:dbl, "测量检出限"=w379:dbl, "测量信号值"=w378:dbl, "线性相关系数"=w377:dbl, "二次多项式系数"=w376:dbl, "标样校准时间"=w375:timestamp, "稀释倍数"=w374:dbl)
                n223 = Bundle By Name(cluster=w389, "测量量程"=w387, "测量精度"=w386, "测量间隔"=w385, "消解温度"=w384, "消解时长"=w383, "空白校准时间"=w382, "曲线截距"=w381, "曲线斜率"=w380, "测量检出限"=w379, "测量信号值"=w378, "线性相关系数"=w377, "二次多项式系数"=w376, "标样校准时间"=w375, "稀释倍数"=w374) -> (w373:T16)
                n224 = global write "CODcr全局变量.vi" "CODCr仪器参数"(w373) -> ()
              }
              frame #1 {
                n225 = call <vilib>:"Application Directory.vi"() -> ("Application Directory"=w403:path)
                n226 = Build Path(base path=w403, name or relative path="data\\sys.ini" ("名称或相对路径")) -> (appended path=w401:path)
                n227 = call <vilib>:"Open Config Data.vi"("configuration file path"=w401) -> ("error out"=w397:errorcluster, "refnum"=w400:T7)  [unwired: 8 in, 1 out]
                n228 = vi-ref "CODCr库.lvlib:CODcr全局变量.vi"() -> (w399:refnum<vi>)
                n229 = call <userlib>:"Write Panel to INI__ogtk.vi"("error in (no error)"=w397, "VI ref"=w399, "refnum"=w400) -> ("error out"=w396:errorcluster, "refnum out"=w398:T7)  [unwired: 7 in]
                n230 = call <vilib>:"Close Config Data.vi"("error in (no error)"=w396, "refnum"=w398) -> ("error out"=w391:errorcluster, "file path"=w390:path)  [unwired: 8 in]
                n231 = Open/Create/Replace File(file path (use dialog)=w390, error in=w391) -> (refnum out=w394:refnum<file>, error out=w395:errorcluster)  [unwired: 4 in, 1 out]
                n232 = Flush File(refnum=w394, error in=w395) -> (refnum out=w393:refnum<file>, error out=w392:errorcluster)
                n233 = Close File(refnum=w393, error in=w392) -> ()  [unwired: 2 out]
              }
            }
          }
        }
      }
      event "打开串口": Value Change {
        n234 = event-data() -> ()  [unwired: 1 in, 6 out]
        n235 = global read "CODcr全局变量.vi" "VISA Resource"() -> (w412:refnum<visa-resource-name>)
        n236 = global read "CODcr全局变量.vi" "PORT"() -> (w406:string)
        n237 = global read "CODcr全局变量.vi" "IP"() -> (w407:string)
        n238 = call "串口配置.vi"("PORT"=w406, "IP"=w407, "请选择串口:"=w412) -> ("PORT 2"=w408:string, "IP 2"=w409:string, "确认 2"=w411:bool, "VISA资源名称 2"=w410:refnum<visa-resource-name>)  [unwired: 5 in]
        n239 = case shown="真" w411 {
          tunnel: w410 -> [_ w415]
          tunnel: w405 -> [_ w417]
          tunnel: w404 -> [_ w416]
          tunnel: w409 -> [_ w414]
          tunnel: w408 -> [_ w413]
          frame False {
          }
          frame True {
            n240 = global write "CODcr全局变量.vi" "VISA Resource"(w415) -> ()
            n241 = global write "CODcr全局变量.vi" "PORT"(w413) -> ()
            n242 = global write "CODcr全局变量.vi" "IP"(w414) -> ()
            n243 = Bundle By Name(cluster=cluster{"命令":string} {"命令"=""} ("元素"), "命令"="启用模块" ("名称（未命名）")) -> (w418:cluster{"命令":string})
            n244 = Enqueue Element(queue=w417, element=w418, error in (no error)=w416) -> ()  [unwired: 1 in, 3 out]
          }
        }
      }
      event "释放串口": Value Change {
        n245 = event-data() -> ()  [unwired: 1 in, 6 out]
        n246 = Two Button Dialog(message="确认是否释放串口，释放串口将导致通信失败！" ("消息")) -> (T button?=w423:bool)  [unwired: 2 in]
        n247 = case shown="真" w423 {
          tunnel: w422 -> [_ w426]
          tunnel: w421 -> [_ w425]
          frame False {
          }
          frame True {
            n248 = Bundle By Name(cluster=cluster{"命令":string} {"命令"=""} ("元素"), "命令"="停用模块" ("名称（未命名）")) -> (w427:cluster{"命令":string})
            n249 = Enqueue Element(queue=w426, element=w427, error in (no error)=w425) -> ()  [unwired: 1 in, 3 out]
          }
        }
      }
      event "MB通信方式选择": Value Change {
        n250 = event-data() -> ()  [unwired: 1 in, 6 out]
        n251 = flat-sequence {
          frame #0 {
            n252 = global write "CODcr全局变量.vi" "MB通信方式选择"("MB通信方式选择") -> ()
          }
          frame #1 {
            n253 = call <vilib>:"Application Directory.vi"() -> ("Application Directory"=w444:path)
            n254 = Build Path(base path=w444, name or relative path="data\\sys.ini" ("名称或相对路径")) -> (appended path=w442:path)
            n255 = call <vilib>:"Open Config Data.vi"("configuration file path"=w442) -> ("error out"=w438:errorcluster, "refnum"=w441:T7)  [unwired: 8 in, 1 out]
            n256 = vi-ref "CODCr库.lvlib:CODcr全局变量.vi"() -> (w440:refnum<vi>)
            n257 = call <userlib>:"Write Panel to INI__ogtk.vi"("error in (no error)"=w438, "VI ref"=w440, "refnum"=w441) -> ("error out"=w437:errorcluster, "refnum out"=w439:T7)  [unwired: 7 in]
            n258 = call <vilib>:"Close Config Data.vi"("error in (no error)"=w437, "refnum"=w439) -> ("error out"=w432:errorcluster, "file path"=w431:path)  [unwired: 8 in]
            n259 = Open/Create/Replace File(file path (use dialog)=w431, error in=w432) -> (refnum out=w435:refnum<file>, error out=w436:errorcluster)  [unwired: 4 in, 1 out]
            n260 = Flush File(refnum=w435, error in=w436) -> (refnum out=w434:refnum<file>, error out=w433:errorcluster)
            n261 = Close File(refnum=w434, error in=w433) -> ()  [unwired: 2 out]
          }
        }
      }
      event "写入消解温度时长": Value Change {
        n262 = event-data() -> ()  [unwired: 1 in, 6 out]
        n263 = local read "消解时长"() -> (w449:u16)
        n264 = local read "消解温度"() -> (w450:u16)
        n265 = Build Array(w450, w449) -> (w448:u16[])
        n266 = call "WordToHex.vi"("WORD"=w448) -> ("数组"=w445:u16[])  [unwired: 10 in]
        n267 = call "CODCrMB_api.vi"("STEP"=enum16{"open", "read", "write", "close"}."write", "values"=w445, "starting address"=u16 4257) -> ()  [unwired: 6 in, 3 out]
      }
      event "校时": Value Change {
        n268 = event-data() -> ()  [unwired: 1 in, 6 out]
        n269 = Get Date/Time In Seconds() -> (seconds since 1Jan1904=w458:timestamp)
        n270 = Build Array(w458) -> (w455:timestamp[])
        n271 = call "DateToHex.vi"("DATE"=w455) -> ("数组"=w454:u16[])  [unwired: 10 in]
        n272 = Insert Into Array(array=u16[] [13] ("values"), index=1 ("索引"), new element=w454) -> (w451:u16[])
        n273 = call "CODCrMB_api.vi"("STEP"=enum16{"open", "read", "write", "close"}."write", "values"=w451, "starting address"=u16 4608) -> ()  [unwired: 6 in, 3 out]
      }
      event "设置": Value Change {
        n274 = event-data() -> ()  [unwired: 1 in, 6 out]
        n275 = property on="窗格" class="Pane"("Origin"=T6 {"Horizontal"=0, "Vertical"=728} ("原点")) -> ()  [unwired: 2 in, 2 out]
        n276 = Bundle By Name(cluster=cluster{"命令":string} {"命令"=""} ("元素"), "命令"="CODCr读取参数" ("名称（未命名）")) -> (w461:cluster{"命令":string})
        n277 = Enqueue Element(queue=w460, element=w461, error in (no error)=w459) -> ()  [unwired: 1 in, 3 out]
      }
      event "返回": Value Change {
        w465 = FALSE ("可见")
        n278 = event-data() -> ()  [unwired: 1 in, 6 out]
        n279 = property on="窗格" class="Pane"("Origin"=T6 {"Horizontal"=0, "Vertical"=0} ("原点")) -> ()  [unwired: 2 in, 2 out]
        n280 = property on="写入消解温度时长" class="Bool"("Visible"=w465) -> ()  [unwired: 2 in, 2 out]
        n281 = property on="释放串口" class="Bool"("Visible"=w465) -> ()  [unwired: 2 in, 2 out]
        n282 = property on="打开串口" class="Bool"("Visible"=w465) -> ()  [unwired: 2 in, 2 out]
        n283 = property on="MB通信方式选择" class="Enum (严格)"("Visible"=w465) -> ()  [unwired: 2 in, 2 out]
      }
      event "曲线斜率K", "曲线截距B", "消解温度", "消解时长": Mouse Down {
        n284 = event-data() -> ("CtlRef"=w469:refnum<vi>)  [unwired: 1 in, 7 out]
        n285 = property class="DigNum"(reference=w469) -> (reference out=w470:refnum<vi>, "Value"=w468:variant)  [unwired: 1 in, 1 out]
        n286 = Variant To Data(Variant=w468) -> (data=w467:sgl)  [unwired: 2 in, 1 out]
        n287 = call "CODCR数字键盘.vi"("OldNumber"=w467) -> ("NewNumber"=w471:sgl)
        n288 = property class="DigNum"(reference=w470, "Value"=w471) -> ()  [unwired: 1 in, 2 out]
      }
      event "隐藏按钮": Value Change {
        w472 = TRUE ("可见")
        n289 = event-data() -> ()  [unwired: 1 in, 6 out]
        n290 = property on="写入消解温度时长" class="Bool"("Visible"=w472) -> ()  [unwired: 2 in, 2 out]
        n291 = property on="释放串口" class="Bool"("Visible"=w472) -> ()  [unwired: 2 in, 2 out]
        n292 = property on="打开串口" class="Bool"("Visible"=w472) -> ()  [unwired: 2 in, 2 out]
        n293 = property on="MB通信方式选择" class="Enum (严格)"("Visible"=w472) -> ()  [unwired: 2 in, 2 out]
      }
    }
  }
  n294 = while {
    tunnel: w20 -> [w474]
    tunnel: w19 -> [w473]
    i -> [w482]
    stop <- FALSE stop-if-true
    n295 = First Call?() -> (First Call?: T/F=w477:bool)
    n296 = case shown="真" w477 {
      tunnel: w474 -> [w486 w491]
      tunnel: w473 -> [w485 w490]
      tunnel: [w486 w489] -> w476
      tunnel: [w485 w488] -> w475
      frame False {
      }
      frame True {
        n297 = Bundle By Name(cluster=cluster{"命令":string} {"命令"=""} ("元素"), "命令"="CODMn读取参数" ("名称（未命名）")) -> (w494:cluster{"命令":string})
        n298 = Enqueue Element(queue=w491, element=w494, timeout in ms (-1)=1000 ("超时毫秒(-1)"), error in (no error)=w490) -> (queue out=w489:refnum<queue>, error out=w488:errorcluster)  [unwired: 1 out]
      }
    }
    n299 = Get Queue Status(queue=w476, error in (no error)=w475) -> (queue out=w480:refnum<queue>, error out=w479:errorcluster, # elements in queue=w481:i32)  [unwired: 1 in, 5 out]
    n300 = Equal To 0?(x=w481) -> (x = 0?=w478:bool)
    n301 = case shown="真" w478 {
      tunnel: w480 -> [_ w496]
      tunnel: w479 -> [_ w495]
      frame False {
      }
      frame True {
        n302 = Bundle By Name(cluster=cluster{"命令":string} {"命令"=""} ("元素"), "命令"="CODCr读取" ("名称（未命名）")) -> (w498:cluster{"命令":string})
        n303 = Enqueue Element(queue=w496, element=w498, timeout in ms (-1)=1000 ("超时毫秒(-1)"), error in (no error)=w495) -> ()  [unwired: 3 out]
      }
    }
    n304 = Wait (ms)(milliseconds to wait=u32 1000 ("等待时间（毫秒）")) -> ()  [unwired: 1 out]
    "主循环次数" <- w482
  }
